vi "LOC subReadWriteVIStringINIKeys(TabControl).vi"(4 "Mode":enum16{"Read", "Write"}(ring), 5 "Section":string, 6 "error in (no error)":errorcluster, 8 "ConfigFileRefnum":T1, 9 "ControlRefnum":refnum<vi>) -> (0 "error out":errorcluster)   [LabVIEW 2020, in "Localization_Tools.lvlib"]
uses:
  Localization_Tools.lvlib
  <vilib>/Utility/config.llb/Config Data RefNum.ctl
  <vilib>/Utility/config.llb/NI_LVConfig.lvlib
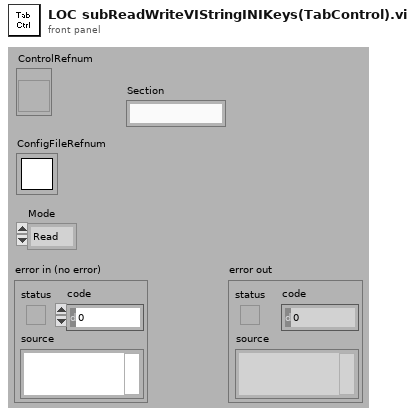
[diagram p1: front panel]
types:
  T1 = typedef "NI_LVConfig.lvlib/Config Data RefNum.ctl" = refnum<k1>
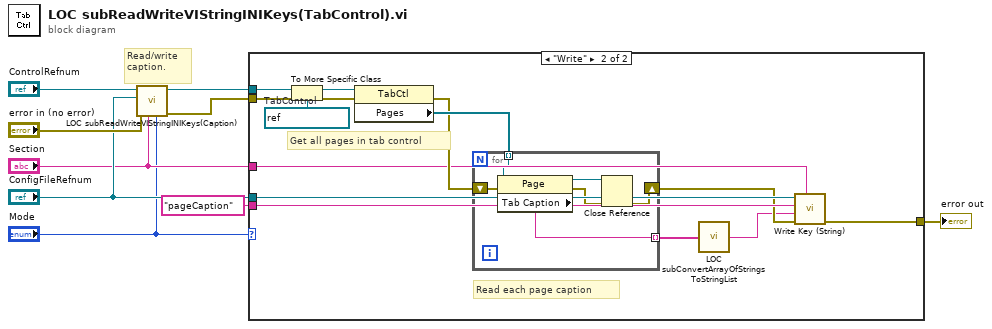
[diagram p0: block diagram]
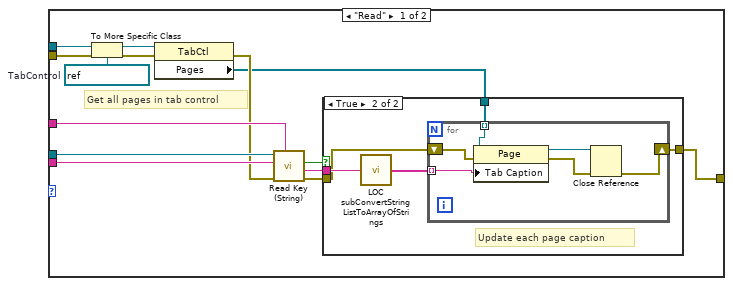
[diagram p2: hidden frame]
diagram:
  # "Read/write\ncaption."
  n1 = call "LOC subReadWriteVIStringINIKeys(Caption).vi"("Mode"="Mode", "Section"="Section", "error in (no error)"="error in (no error)", "ConfigFileRefnum"="ConfigFileRefnum", "ControlRefnum"="ControlRefnum") -> ("error out"=w4:errorcluster, "dup ControlRefnum"=w6:refnum<vi>)  [unwired: 3 in]
  n2 = case shown="\"Write\"" "Mode" {
    tunnel: w6 -> [w18 w47]
    tunnel: w4 -> [w17 w46]
    tunnel: "ConfigFileRefnum" -> [w23 w42]
    tunnel: "Section" -> [w22 w40]
    tunnel: "pageCaption" ("key") -> [w21 w41]
    tunnel: [w13 w38] -> w8
    frame "Read" {
      w20 = refnum<vi> refnum  # TabControl
      # "Get all pages in tab control"
      n3 = To More Specific Class(target class=w20, reference=w18, error in=w17) -> (specific class reference=w19:refnum<vi>, error out=w16:errorcluster)
      n4 = property class="TabCtl"(reference=w19, error in=w16) -> (error out=w15:errorcluster, "Pages"=w14:refnum<vi>[])  [unwired: 1 out]
      n5 = call <vilib>:"Read Key (String).vi"("section"=w22, "error in (no error)"=w15, "key"=w21, "refnum"=w23) -> ("error out"=w11:errorcluster, "value"=w12:string, "found?"=w10:bool)  [unwired: 4 in, 1 out]
      n6 = case shown="True" w10 {
        tunnel: w14 -> [_ w29]
        tunnel: [w24 w28] -> w13
        tunnel: w12 -> [_ w27]
        tunnel: w11 -> [w24 w25]
        frame False {
        }
        frame True {
          # "Update each page caption"
          n7 = call "LOC subConvertStringListToArrayOfStrings.vi"("InputString"=w27) -> ("OutputArray"=w26:string[])
          n8 = for {
            tunnel: w29 -> [w33] mode=indexing
            shift-right: [w32] -> w28
            shift-left: w25 -> [w31]
            tunnel: w26 -> [w30] mode=indexing
            n9 = property class="Page"(reference=w33, error in=w31, "Tab Caption"=w30) -> (reference out=w35:refnum<vi>, error out=w34:errorcluster)
            n10 = Close Reference(reference=w35, error in (no error)=w34) -> (error out=w32:errorcluster)
          }
        }
      }
    }
    frame "Write" {
      w49 = refnum<vi> refnum  # TabControl
      # "Get all pages in tab control"
      # "Read each page caption"
      n11 = To More Specific Class(target class=w49, reference=w47, error in=w46) -> (specific class reference=w48:refnum<vi>, error out=w45:errorcluster)
      n12 = property class="TabCtl"(reference=w48, error in=w45) -> (error out=w43:errorcluster, "Pages"=w44:refnum<vi>[])  [unwired: 1 out]
      n13 = for {
        tunnel: w44 -> [w53] mode=indexing
        shift-right: [w52] -> w39
        shift-left: w43 -> [w51]
        tunnel: [w50] -> w37 mode=indexing
        n14 = property class="Page"(reference=w53, error in=w51) -> (reference out=w55:refnum<vi>, error out=w54:errorcluster, "Tab Caption"=w50:string)
        n15 = Close Reference(reference=w55, error in (no error)=w54) -> (error out=w52:errorcluster)
      }
      n16 = call "LOC subConvertArrayOfStringsToStringList.vi"("InputArray"=w37) -> ("OutputString"=w36:string)
      n17 = call <vilib>:"Write Key (String).vi"("section"=w40, "error in (no error)"=w39, "value"=w36, "key"=w41, "refnum"=w42) -> ("error out"=w38:errorcluster)  [unwired: 4 in, 2 out]
    }
  }
  "error out" <- w8
